vi "RSZVB Get Font Size.vi"(8 "error in (no error)":errorcluster {"code" format="%.0x"}, 11 "VISA session":refnum<visa-resource-name>) -> (0 "error out":errorcluster {"code" format="%.0x"}, 1 "Font Size":i32, 3 "dup VISA session":refnum<visa-resource-name>)   [LabVIEW 2011]
doc: "This VI returns the size of the fonts in the diagram on a relative scale. \n\nRemote-control command(s):\nDISPlay:RFSize?"
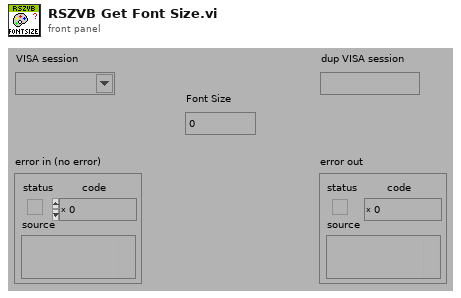
[diagram p1: front panel]
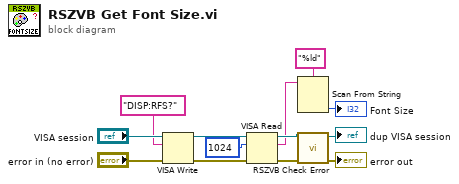
[diagram p0: block diagram]
diagram:
  n1 = VISA Write(VISA resource name="VISA session", write buffer="DISP:RFS?", error in (no error)="error in (no error)") -> (VISA resource name out=w6:refnum<visa-resource-name>, error out=w5:errorcluster)  [unwired: 1 out]
  n2 = VISA Read(VISA resource name=w6, byte count=u32 1024 ("byte count (0)"), error in (no error)=w5) -> (VISA resource name out=w7:refnum<visa-resource-name>, read buffer=w3:string, error out=w8:errorcluster)  [unwired: 1 out]
  n3 = Scan From String(format string="%ld", input string=w3) -> (output 1=→"Font Size":i32)  [unwired: 3 in, 3 out]
  n4 = call "RSZVB Check Error.vi"("error in (no error)"=w8, "VISA session"=w7) -> ("error out"=→"error out":errorcluster, "dup VISA session"=→"dup VISA session":refnum<visa-resource-name>)  [unwired: 8 in]
